vi "Event Self Alias.vi"(11 "Base Event jettl in":refnum<class "Base Event jettl.lvclass">) -> (2 "Event Self Alias":string)   [LabVIEW 2021, in "jettl.lvlib" / "Base Event jettl.lvlib" / "Base Event jettl.lvclass"]
uses:
  Base Event jettl.lvclass
  Base Event jettl.lvclass/Base Event jettl.ctl
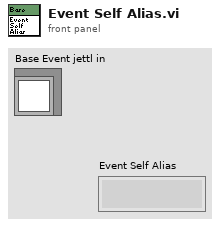
[diagram p1: front panel]
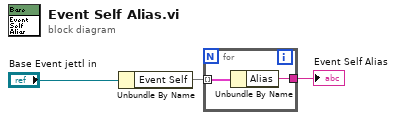
[diagram p0: block diagram]
diagram:
  n1 = Unbundle By Name("Base Event jettl in") -> ("Event Self"=w1:map{string, refnum<data-value>})
  n2 = for {
    tunnel: w1 -> [w5] mode=indexing
    tunnel: [w4] -> w2
    n3 = Unbundle By Name(w5) -> ("Alias"=w4:string)
  }
  "Event Self Alias" <- w2
